vi "测量数据区.vi"(11 "数组":u16[](array[numeric]) format="%04xH") -> (3 "测量数据区":T1 {"单位" items=["ug/L", "mg/L", "ppm", "mg/m3", "cm", "ppb", "ug/m3", "%", "nmol/mol", "umol/mol", "MPN/L", "MPN/100ml", "ng/m3", "NTU", "无量纲", "ms/cm", "us/cm", "℃", "mV", "万个/L"]})   [LabVIEW 2016, in "总磷.lvlib"]
panel:
  # "共占用95 WORD"
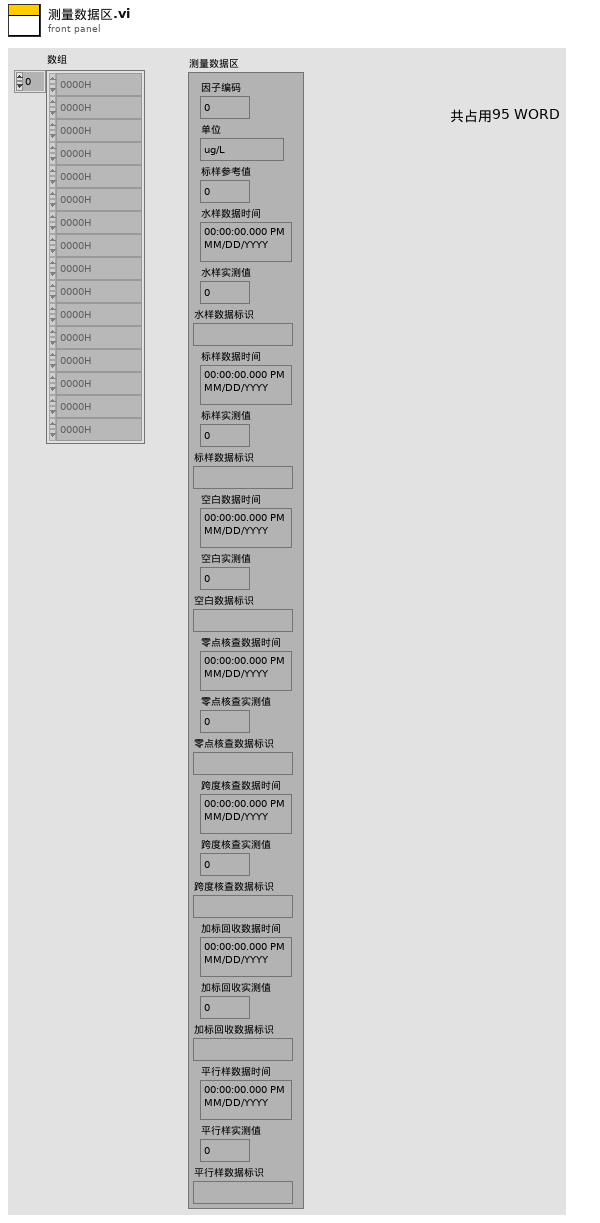
[diagram p1: front panel]
types:
  T1 = cluster{"因子编码":u32, "单位":u16, "标样参考值":sgl, "水样数据时间":timestamp, "水样实测值":sgl, "水样数据标识":string, "标样数据时间":timestamp, "标样实测值":sgl, "标样数据标识":string, "空白数据时间":timestamp, "空白实测值":sgl, "空白数据标识":string, "零点核查数据时间":timestamp, "零点核查实测值":sgl, "零点核查数据标识":string, "跨度核查数据时间":timestamp, "跨度核查实测值":sgl, "跨度核查数据标识":string, "加标回收数据时间":timestamp, "加标回收实测值":sgl, "加标回收数据标识":string, "平行样数据时间":timestamp, "平行样实测值":sgl, "平行样数据标识":string}
  T2 = cluster{"DWORD":i32, "WORD":u16, "FLOAT":sgl, "time stamp":timestamp, "数值":sgl, "string":string, "time stamp":timestamp, "数值":sgl, "string":string, "time stamp":timestamp, "数值":sgl, "string":string, "time stamp":timestamp, "数值":sgl, "string":string, "time stamp":timestamp, "数值":sgl, "string":string, "time stamp":timestamp, "数值":sgl, "string":string, "time stamp":timestamp, "数值":sgl, "string":string}
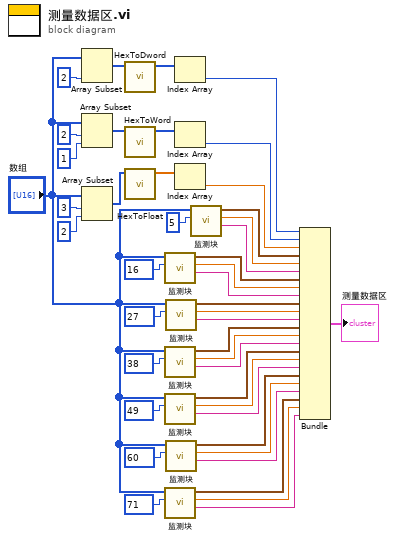
[diagram p0: block diagram]
diagram:
  n1 = Array Subset(array="数组", length=2 ("长度")) -> (w44:u16[])  [unwired: 1 in]
  n2 = Array Subset(array="数组", index=2 ("索引"), length=1 ("长度")) -> (w39:u16[])
  n3 = Array Subset(array="数组", index=3 ("索引"), length=2 ("长度")) -> (w34:u16[])
  n4 = call "HexToDword.vi"("数组"=w44) -> ("DWORD"=w42:i32[])  [unwired: 10 in]
  n5 = call "HexToWord.vi"("数组"=w39) -> ("WORD"=w38:u16[])  [unwired: 10 in]
  n6 = call "HexToFloat.vi"("数组"=w34) -> ("FLOAT"=w33:sgl[])  [unwired: 10 in]
  n7 = call "监测块.vi"("索引"=16, "数组"="数组") -> ("string"=w24:string, "数值"=w25:sgl, "time stamp"=w26:timestamp)  [unwired: 7 in]
  n8 = call "监测块.vi"("索引"=38, "数组"="数组") -> ("string"=w16:string, "数值"=w17:sgl, "time stamp"=w18:timestamp)  [unwired: 7 in]
  n9 = call "监测块.vi"("索引"=49, "数组"="数组") -> ("string"=w12:string, "数值"=w13:sgl, "time stamp"=w14:timestamp)  [unwired: 7 in]
  n10 = call "监测块.vi"("索引"=71, "数组"="数组") -> ("string"=w4:string, "数值"=w5:sgl, "time stamp"=w6:timestamp)  [unwired: 7 in]
  n11 = call "监测块.vi"("索引"=27, "数组"="数组") -> ("string"=w20:string, "数值"=w21:sgl, "time stamp"=w22:timestamp)  [unwired: 7 in]
  n12 = call "监测块.vi"("索引"=60, "数组"="数组") -> ("string"=w8:string, "数值"=w9:sgl, "time stamp"=w10:timestamp)  [unwired: 7 in]
  n13 = Index Array(array=w42) -> (element=w2:i32)  [unwired: 1 in]
  n14 = Index Array(array=w38) -> (element=w37:u16)  [unwired: 1 in]
  n15 = Index Array(array=w33) -> (element=w32:sgl)  [unwired: 1 in]
  n16 = call "监测块.vi"("索引"=5, "数组"="数组") -> ("string"=w29:string, "数值"=w30:sgl, "time stamp"=w31:timestamp)  [unwired: 7 in]
  n17 = Bundle("DWORD"=w2, "WORD"=w37, "FLOAT"=w32, "time stamp"=w31, "数值"=w30, "string"=w29, "time stamp"=w26, "数值"=w25, "string"=w24, "time stamp"=w22, "数值"=w21, "string"=w20, "time stamp"=w18, "数值"=w17, "string"=w16, "time stamp"=w14, "数值"=w13, "string"=w12, "time stamp"=w10, "数值"=w9, "string"=w8, "time stamp"=w6, "数值"=w5, "string"=w4) -> (→"测量数据区":T2)  [unwired: 1 in]
